vi "Cluster.vi"(8 "error in":errorcluster, 10 "Action":enum16{"Write", "Read"}(ring), 11 "Cluster":T1 {"Green-Red" step=1 scale=0.0..100.0; "Blue" step=1 scale=0.0..100.0; "Violet" step=1 scale=0.0..100.0}) -> (0 "error out":errorcluster, 3 "Cluster":T1 {"Green-Red" step=1 scale=0.0..100.0; "Blue" step=1 scale=0.0..100.0; "Violet" step=1 scale=0.0..100.0})   [LabVIEW 2025]
doc: "Functional Global Variable:\n- Write the value into the memory \nor\n- Read the value from the memory"
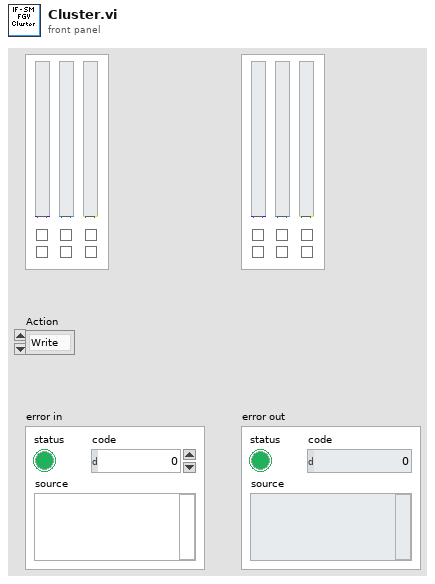
[diagram p1: front panel]
types:
  T1 = cluster{"Violet":u8, "Blue":u8, "Green-Red":u8, "A(S)Selected/(N)Unselected":bool, "B(S)Selected/(N)Unselected":bool, "C(S)Selected/(N)Unselected":bool, "A(N)ON/(F)OFF":bool, "(N)ON/(F)OFF":bool, "C(N)ON/(F)OFF":bool}
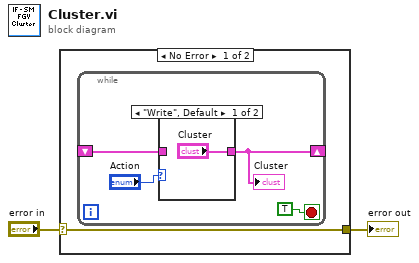
[diagram p0: block diagram]
diagram:
  n1 = case shown="No Error" "error in" {
    selector: "error in" -> [w3 w10]
    tunnel: [w3 w10] -> w1
    frame No Error {
      n2 = while {
        shift-right: [w4] -> _
        shift-left: _ -> [w5]
        stop <- TRUE stop-if-true
        n3 = case shown="\"Write\", Default" "Action" {
          tunnel: w5 -> [_ w9]
          tunnel: ["Cluster" w9] -> w4
          frame "Write", Default {
          }
          frame "Read" {
          }
        }
        "Cluster" <- w4
      }
    }
    frame Error {
    }
  }
  "error out" <- w1
